vi "plot_run.vi"(0 "xValues":i32, 1 "yValues":i32, 2 "File Path":path, 3 "xName":string, 4 "yName":string) -> ()   [LabVIEW 2019]
uses:
  <vilib>/Analysis/Matrix/Numeric/Conversions/Array To Matrix - RA2.vi
  <vilib>/Analysis/Matrix/Numeric/Conversions/Matrix To Array - RM.vi
  <vilib>/Analysis/Matrix/NI_Matrix.lvlib
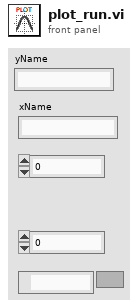
[diagram p1: front panel]
types:
  T1 = typedef "NI_Matrix.lvlib/RealMatrix.ctl" = dbl[][]
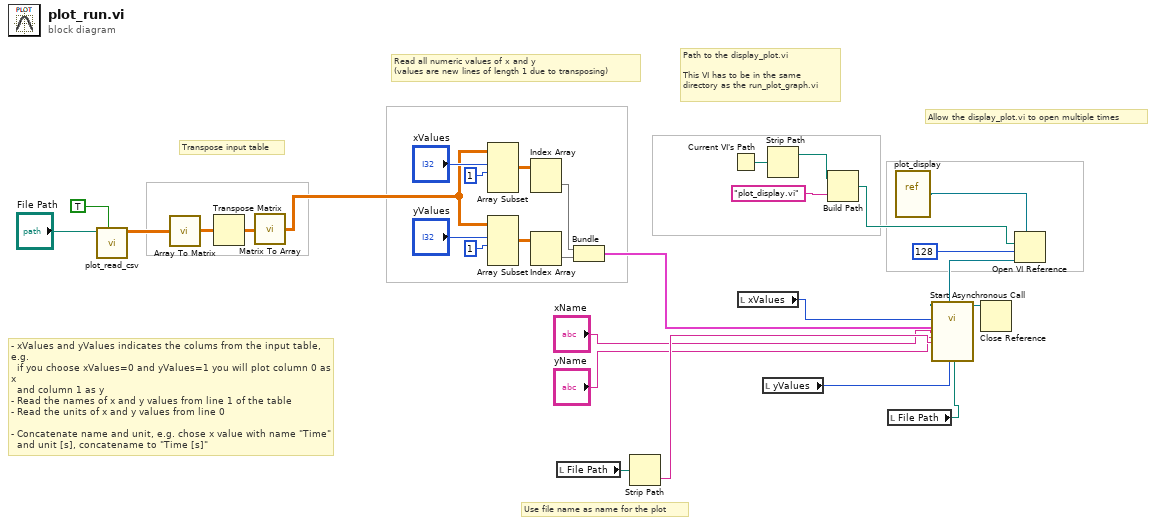
[diagram p0: block diagram]
diagram:
  # "Path to the display_plot.vi\n\nThis VI has to be in the same \ndirectory as the run_plot_graph.vi"
  # "Allow the display_plot.vi to open multiple times"
  # "Use file name as name for the plot"
  # "Read all numeric values of x and y\n(values are new lines of length 1 due to transposing)"
  # "Transpose input table"
  # "- xValues and yValues indicates the colums from the input table, e.g.\n  if you choose xValues=0 and yValues=1 you will plot column 0 as x \n  and column 1 as y\n- Read the names of x and y values from line 1 of the table\n- Read the units of x and y values from line 0\n\n- Concatenate name and unit, e.g. chose x value with name \"Time\"\n  and unit [s], concatename to \"Time [s]\""
  n1 = call "plot_read_csv.vi"("Read"=TRUE, "Read File:"="File Path") -> ("File Data"=w19:T1)  [unwired: 9 in]
  n2 = call-poly <vilib>:"Array To Matrix.vi"("Real 2D Array"=w19) -> ("Real Matrix"=w28:T1)
  n3 = Transpose Matrix(1:w28) -> (0:w29:T1)
  n4 = call-poly <vilib>:"Matrix To Array.vi"("Real Matrix"=w29) -> ("Real 2D Array"=w25:dbl[][])
  n5 = Array Subset(array=w25, index (row)="xValues", length (row)=1 ("length")) -> (w24:dbl[][])  [unwired: 2 in]
  n6 = Array Subset(array=w25, index (row)="yValues", length (row)=1 ("length")) -> (w22:dbl[][])  [unwired: 2 in]
  n7 = Index Array(array=w24) -> (element=w23:dbl[])  [unwired: 2 in]
  n8 = Index Array(array=w22) -> (element=w21:dbl[])  [unwired: 2 in]
  n9 = local read "File Path"() -> (w15:path)
  n10 = Bundle(w23, w21) -> (w7:cluster{dbl[], dbl[]})  [unwired: 1 in]
  n11 = Strip Path(path=w15) -> (name=w6:string)  [unwired: 1 out]
  n12 = Current VI's Path() -> (path=w13:path)
  n13 = local read "xValues"() -> (w3:i32)
  n14 = local read "yValues"() -> (w2:i32)
  n15 = Strip Path(path=w13) -> (stripped path=w12:path)  [unwired: 1 out]
  n16 = Build Path(base path=w12, name or relative path="plot_display.vi" ("string")) -> (appended path=w11:path)
  n17 = local read "File Path"() -> (w1:path)
  n18 = vi-ref "plot_display.vi"() -> (w8:refnum<vi>)
  n19 = Open VI Reference(type specifier VI Refnum (for type only)=w8, vi path=w11, options=128) -> (vi reference=w9:refnum<vi>)  [unwired: 3 in, 1 out]
  n20 = call-by-ref "Start Asynchronous Call"(reference=w9, "Input Data"=w7, "X Scale.Name Label.Text"="xName", "Y Scale.Name Label.Text"="yName", "FileName"=w6, "xValues"=w3, "yValues"=w2, "File Path"=w1) -> (reference out=w10:refnum<vi>)  [unwired: 14 in, 1 out]
  n21 = Close Reference(reference=w10) -> ()  [unwired: 1 in, 1 out]
